vi "Example XYGraph Plot Hi-Lite.vi"() -> ()   [LabVIEW 2020]
uses:
  Graph Extensions.lvlib
panel:
  in  "Plot2":bool
  in  "Plot1":bool
  out "XY Graph":cluster{dbl[], dbl[]}[](graph)
  # "Instructions: Move the mouse over the graphs, and adjust any of the options at the right. to see the effect."
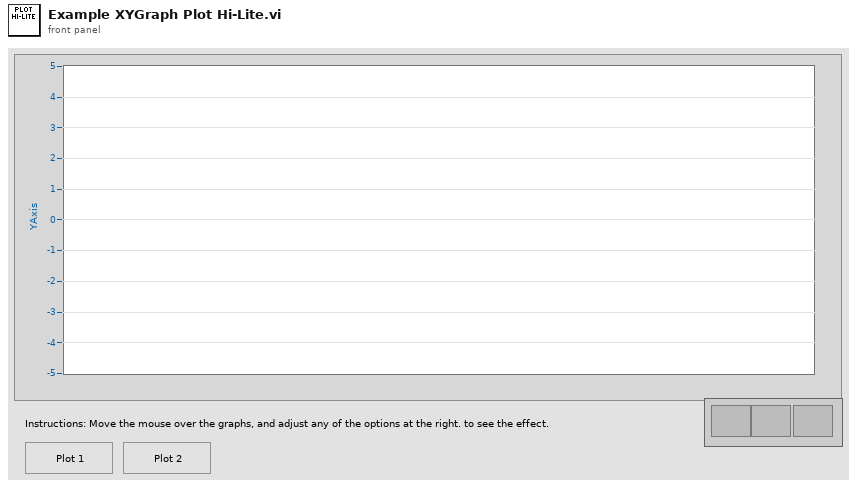
[diagram p1: front panel]
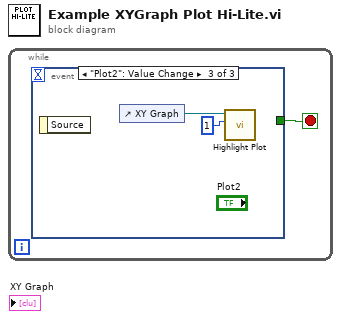
[diagram p0: block diagram]
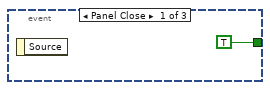
[diagram p2: hidden frame]
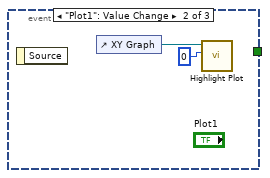
[diagram p3: hidden frame]
diagram:
  n1 = while {
    stop <- w1 stop-if-true
    n2 = event shown="[2] \"Plot2\": Value Change" {
      selector: _ -> [_ _ _]
      dyn-events: _ -> [_ _ _]
      timeout: _ -> [_ _ _]
      tunnel: [TRUE _ _] -> w1
      event Panel Close {
        n3 = event-data() -> ()  [unwired: 1 in, 1 out]
      }
      event "Plot1": Value Change {
        n4 = event-data() -> ()  [unwired: 1 in, 1 out]
        n5 = control-ref of="XY Graph"() -> (w4:refnum<vi>)
        n6 = call "Highlight Plot.vi"("PlotNum"=0, "XYGraph in"=w4) -> ()  [unwired: 10 in]
      }
      event "Plot2": Value Change {
        n7 = event-data() -> ()  [unwired: 1 in, 1 out]
        n8 = control-ref of="XY Graph"() -> (w6:refnum<vi>)
        n9 = call "Highlight Plot.vi"("PlotNum"=1, "XYGraph in"=w6) -> ()  [unwired: 10 in]
      }
    }
  }
